vi "day1 Part Two.vi"() -> ()   [LabVIEW 2025]
panel:
  out "Array 2":i32[](array[numeric])
  out "Array":i32[](array[numeric])
  in  "Test":bool
  out "result":i32
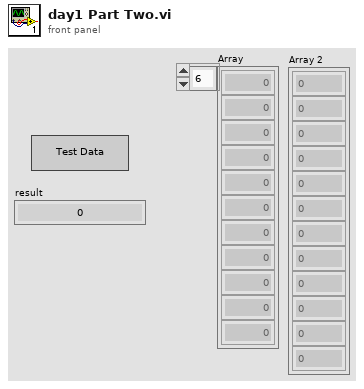
[diagram p1: front panel]
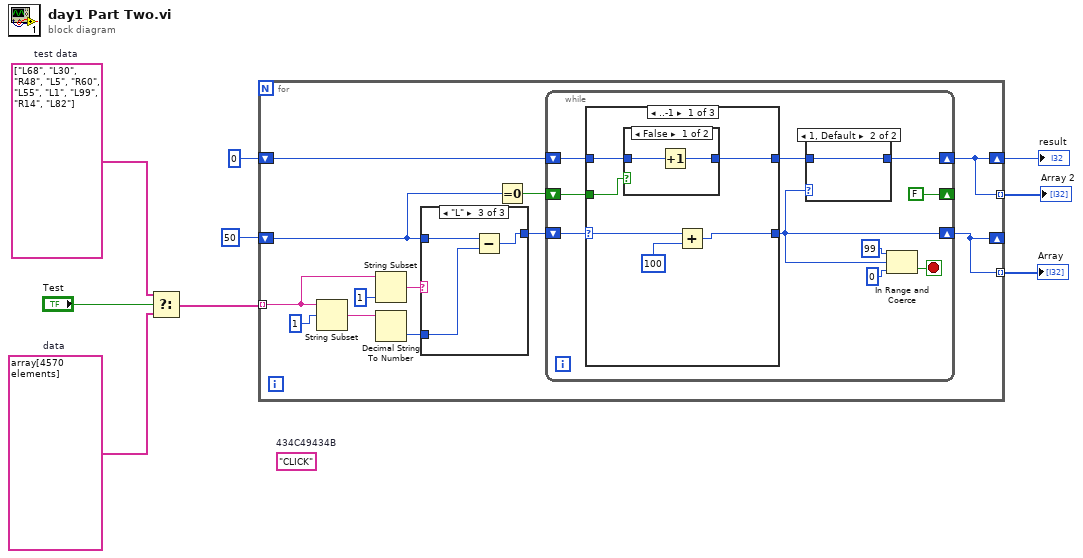
[diagram p0: block diagram]
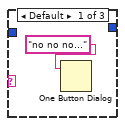
[diagram p2: hidden frame]
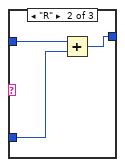
[diagram p3: hidden frame]
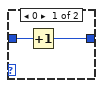
[diagram p4: hidden frame]
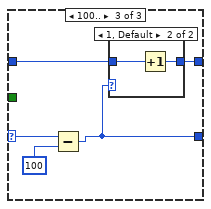
[diagram p7: hidden frame]
diagram:
  w1 = string[] ["L68", "L30", "R48", "L5", "R60", "L55", "L1", "L99", "R14", "L82"]  # test data
  (unwired) "CLICK"  # 434C49434B
  w4 = string[] array[4570 elements]  # data
  n1 = Select(t=w1, s="Test", f=w4) -> (s? t:f=w7:string[])
  n2 = for {
    tunnel: w7 -> [w19] mode=indexing
    shift-right: [w14] -> _
    shift-left: 50 -> [w10]
    shift-right: [w12] -> w8
    shift-left: 0 -> [w13]
    tunnel: [w14] -> w5 mode=indexing
    tunnel: [w12] -> w3 mode=indexing
    n3 = String Subset(string=w19, offset (0)=1) -> (substring=w20:string)  [unwired: 1 in]
    n4 = String Subset(string=w19, length (rest)=1 ("length (rest)")) -> (substring=w18:string)  [unwired: 1 in]
    n5 = Decimal String To Number(string=w20) -> (number=w16:i32)  [unwired: 2 in, 1 out]
    n6 = case shown="\"L\"" w18 {
      tunnel: w16 -> [_ w25 w28]
      tunnel: [_ w24 w27] -> w15
      tunnel: w10 -> [_ w23 w26]
      frame Default {
        n7 = One Button Dialog(message="no no no...") -> ()  [unwired: 1 in, 1 out]
      }
      frame "R" {
        n8 = Add(x=w23, y=w25) -> (x+y=w24:i32)
      }
      frame "L" {
        n9 = Subtract(x=w26, y=w28) -> (x-y=w27:i32)
      }
    }
    n10 = Equal To 0?(x=w10) -> (x = 0?=w11:bool)
    n11 = while {
      shift-right: [w31] -> w14
      shift-left: w15 -> [w38]
      shift-right: [w29] -> w12
      shift-left: w13 -> [w34]
      shift-right: [FALSE] -> _
      shift-left: w11 -> [w33]
      stop <- w37 stop-if-true
      n12 = case shown="..-1" w38 {
        selector: w38 -> [w46 w52 w57]
        tunnel: [w43 w52 w53] -> w31
        tunnel: w34 -> [w47 w51 w55]
        tunnel: w33 -> [w44 _ _]
        tunnel: [w42 w51 w54] -> w30
        frame ..-1 {
          n13 = case shown="False" w44 {
            tunnel: w47 -> [w49 w50]
            tunnel: [w48 w50] -> w42
            frame False {
              n14 = Increment(x=w49) -> (x+1=w48:i32)
            }
            frame True {
            }
          }
          n15 = Add(x=w46, y=100) -> (x+y=w43:i32)
        }
        frame Default {
        }
        frame 100.. {
          n16 = Subtract(x=w57, y=100) -> (x-y=w53:i32)
          n17 = case shown="1, Default" w53 {
            tunnel: w55 -> [w58 w60]
            tunnel: [w58 w59] -> w54
            frame 0 {
            }
            frame 1, Default {
              n18 = Increment(x=w60) -> (x+1=w59:i32)
            }
          }
        }
      }
      n19 = case shown="1, Default" w31 {
        tunnel: w30 -> [w40 w41]
        tunnel: [w39 w41] -> w29
        frame 0 {
          n20 = Increment(x=w40) -> (x+1=w39:i32)
        }
        frame 1, Default {
        }
      }
      n21 = In Range and Coerce(upper limit=99, x=w31, lower limit=0) -> (In Range?=w37:bool)  [unwired: 1 out]
    }
  }
  "result" <- w8
  "Array" <- w5
  "Array 2" <- w3
